vi "Gyro Readings.vi"() -> ()   [LabVIEW 2017]
uses:
  PowerUp2018-LabVIEW-Practice/Team HoneoyeRobotics/FRC2018-master/RobotCode/Framework/Robot Global Data.vi
panel:
  in  "GyroReset":bool
  out "GyroHeading":dbl
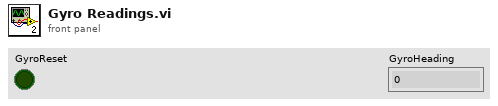
[diagram p1: front panel]
types:
  T1 = typedef "WPI_GyroDevRef.ctl" = cluster{"DevStatus":errorcluster, "Analog Channel":T2, "Gain (VoltsPerDegree/Second)":dbl, "Gyro Type":enum16{"Analog", "XRS450"}, "Handle":i32, "SPI Bus":T3, "Device Found":bool, "Sample Rate":dbl, "Calibrate On Open":bool, "Offset":dbl}
  T2 = typedef "FPGA_AIChannel.ctl" = enum8{"AI 0", "AI 1", "AI 2", "AI 3", "AI MXP 0", "AI MXP 1", "AI MXP 2", "AI MXP 3", "Invalid"}
  T3 = typedef "spi_bus.ctl" = enum16{"SPI On-Board, CS0", "SPI On-Board, CS1", "SPI On-Board, CS2", "SPI On-Board, CS3", "SPI MXP", "Invalid"}
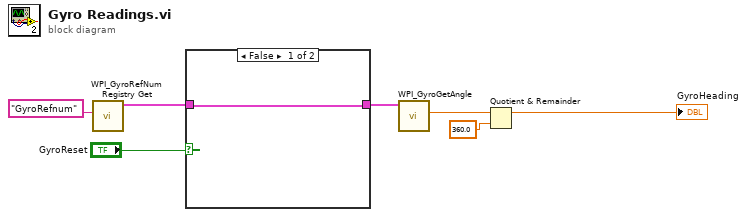
[diagram p0: block diagram]
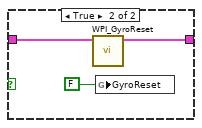
[diagram p2: hidden frame]
diagram:
  n1 = call <vilib>:"WPI_GyroRefNum Registry Get.vi"("refnum name"="GyroRefnum") -> ("GyroDevRef"=w3:T1)  [unwired: 9 in, 1 out]
  n2 = case shown="False" "GyroReset" {
    tunnel: [w8 w10] -> w4
    tunnel: w3 -> [w8 w9]
    frame False {
    }
    frame True {
      n3 = call <vilib>:"WPI_GyroReset.vi"("GyroDevRef"=w9) -> ("GyroDevRef"=w10:T1)  [unwired: 9 in, 1 out]
      n4 = global write "Robot Global Data.vi" "GyroReset"(FALSE ("GyroReset")) -> ()
    }
  }
  n5 = call <vilib>:"WPI_GyroGetAngle.vi"("GyroDevRef"=w4) -> ("Angle"=w5:dbl)  [unwired: 6 in, 4 out]
  n6 = Quotient & Remainder(x=w5, y=360.0) -> (x-y*floor(x/y)=→"GyroHeading":dbl)  [unwired: 1 out]
